vi "autoalignv3.vi"(10 "target":dbl=-0.7824258804321289) -> (2 "rotation":dbl)   [LabVIEW 2020]
uses:
  <vilib>/addons/control/pid/pid.llb/PID (DBL).vi
  <vilib>/addons/control/pid/NI_PID_pid.lvlib
panel:
  in  "PID gains":T1={"proportional gain (Kc)"=0.033, "integral time (Ti, min)"=0.0, "derivative time (Td, min)"=0.0} {"derivative time (Td, min)" format="%.10f"; "integral time (Ti, min)" format="%.10f"; "proportional gain (Kc)" format="%.10f"}
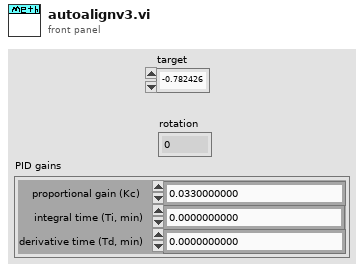
[diagram p1: front panel]
types:
  T1 = cluster{"proportional gain (Kc)":dbl, "integral time (Ti, min)":dbl, "derivative time (Td, min)":dbl}
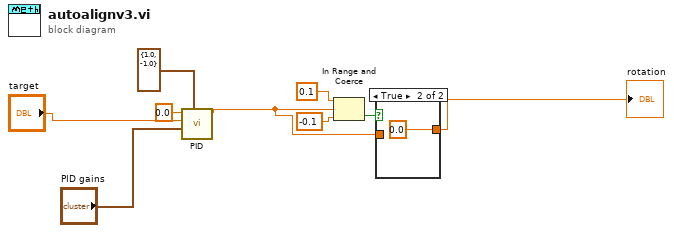
[diagram p0: block diagram]
diagram:
  n1 = call-poly <vilib>:"PID.vi"("output range"=cluster{"output high":dbl, "output low":dbl} {"output high"=1.0, "output low"=-1.0}, "PID gains"="PID gains", "process variable"="target", "setpoint"=0.0) -> ("output"=w2:dbl)  [unwired: 6 in, 1 out]
  n2 = In Range and Coerce(upper limit=0.1, x=w2, lower limit=-0.1) -> (In Range?=w5:bool)  [unwired: 1 out]
  n3 = case shown="True" w5 {
    tunnel: [w10 0.0 ("upper limit")] -> w1
    tunnel: w2 -> [w10 _]
    frame False {
    }
    frame True {
    }
  }
  "rotation" <- w1
